vi "Terminal_Lubricate_Unit_Display.vi"   [LabVIEW 2014]
types:
  T1 = cluster{"径向油缸加载压力":u16, "轴向油缸加载压力":u16, "油箱1油液温度":u16, "润滑油温度":u16, "油箱2油液温度":u16, "试验轴承供油压力":u16, "试验轴承供油流量":u16, "陪试轴承供油流量":u16, "陪试轴承供油压力":u16, "陪试轴承供油温度":u16, "液压子系统状态字":cluster{"加载单元":cluster{"供油过滤器堵塞报警":bool, "回油过滤器堵塞报警":bool, "液位过高报警":bool, "液位过低报警":bool}, "试验轴承单元":cluster{"加热装置异常报警":bool, "油箱1液位过高报警":bool, "油箱1液位过低报警":bool, "油箱2液位过高报警":bool, "油箱2液位过低报警":bool, "供油过滤器堵塞报警":bool, "循环回路过滤器堵塞报警":bool, "回油过滤器堵塞报警":bool}, "陪试轴承单元":cluster{"供油过滤器1堵塞报警":bool, "供油过滤器2堵塞报警":bool, "回油过滤器堵塞报警":bool, "油箱液位过高报警":bool, "油箱液位过低报警":bool}}}
  T2 = cluster{"加热装置异常报警":bool, "油箱1液位过高报警":bool, "油箱1液位过低报警":bool, "油箱2液位过高报警":bool, "油箱2液位过低报警":bool, "供油过滤器堵塞报警":bool, "循环回路过滤器堵塞报警":bool, "回油过滤器堵塞报警":bool}
  T3 = cluster{cluster{sgl, sgl, "油箱1油液温度":u16}, cluster{sgl, sgl, "润滑油温度":u16}, cluster{sgl, sgl, "油箱2油液温度":u16}, cluster{sgl, sgl, "试验轴承供油压力":u16}, cluster{sgl, sgl, "试验轴承供油流量":u16}, "试验轴承单元":cluster{"加热装置异常报警":bool, "油箱1液位过高报警":bool, "油箱1液位过低报警":bool, "油箱2液位过高报警":bool, "油箱2液位过低报警":bool, "供油过滤器堵塞报警":bool, "循环回路过滤器堵塞报警":bool, "回油过滤器堵塞报警":bool}}
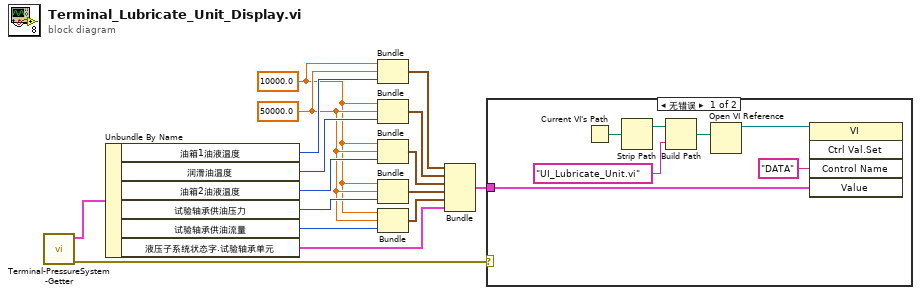
[diagram p0: block diagram]
diagram:
  w10 = sgl 50000.0
  w2 = sgl 10000.0
  n1 = call "Terminal-PressureSystem-Getter.vi"() -> ("error out"=w3:errorcluster, "设备信息"=w16:T1)  [unwired: 10 in]
  n2 = Unbundle By Name(w16) -> ("油箱1油液温度"=w15:u16, "润滑油温度"=w14:u16, "油箱2油液温度"=w13:u16, "试验轴承供油压力"=w12:u16, "试验轴承供油流量"=w11:u16, "液压子系统状态字.试验轴承单元"=w5:T2)
  n3 = Bundle(w2, w10, "油箱1油液温度"=w15) -> (w1:cluster{sgl, sgl, "油箱1油液温度":u16})  [unwired: 1 in]
  n4 = Bundle(w2, w10, "润滑油温度"=w14) -> (w9:cluster{sgl, sgl, "润滑油温度":u16})  [unwired: 1 in]
  n5 = Bundle(w2, w10, "油箱2油液温度"=w13) -> (w8:cluster{sgl, sgl, "油箱2油液温度":u16})  [unwired: 1 in]
  n6 = Bundle(w2, w10, "试验轴承供油压力"=w12) -> (w7:cluster{sgl, sgl, "试验轴承供油压力":u16})  [unwired: 1 in]
  n7 = Bundle(w2, w10, "试验轴承供油流量"=w11) -> (w6:cluster{sgl, sgl, "试验轴承供油流量":u16})  [unwired: 1 in]
  n8 = Bundle(w1, w9, w8, w7, w6, "试验轴承单元"=w5) -> (w4:T3)  [unwired: 1 in]
  n9 = case shown="无错误" w3 {
    tunnel: w4 -> [w17 _]
    frame No Error {
      n10 = Current VI's Path() -> (path=w21:path)
      n11 = Strip Path(path=w21) -> (stripped path=w22:path)  [unwired: 1 out]
      n12 = Build Path(base path=w22, name or relative path="UI_Lubricate_Unit.vi") -> (appended path=w19:path)
      n13 = Open VI Reference(vi path=w19) -> (vi reference=w18:refnum<vi>)  [unwired: 5 in, 1 out]
      n14 = invoke class="VI" method="Ctrl Val.Set"(reference=w18, "Control Name"="DATA", "Value"=w17) -> ()  [unwired: 2 in, 5 out]
    }
    frame Error {
    }
  }
